vi "Delete DVR Entry for DeviceID.vi"(10 "DVR Array":refnum<data-value>[](array[refnum]), 11 "DeviceID":T1) -> ()   [LabVIEW 2018]
uses:
  <vilib>/ORNL/CSEISMIC DDS/CSEISMIC DDS Base/Data Types/Controls/DeviceID.ctl
  <vilib>/ORNL/CSEISMIC DDS/CSEISMIC DDS Base/CSEISMIC DDS.lvclass
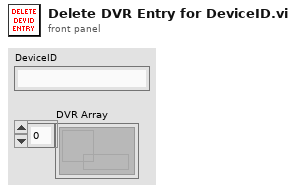
[diagram p1: front panel]
types:
  T1 = typedef "CSEISMIC DDS.lvlib/CSEISMIC DDS.lvclass/DeviceID.ctl" = string
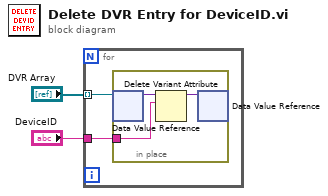
[diagram p0: block diagram]
diagram:
  n1 = for {
    tunnel: "DVR Array" -> [w4] mode=indexing
    tunnel: "DeviceID" -> [w3]
    n2 = in-place {
      in-place-border: w3 -> [w6]
      n3 = in-place-dvr #1(w4) -> (w7:variant)  [unwired: 1 out]
      n4 = Delete Variant Attribute(6:w6, 7:w7) -> (3:w5:variant)  [unwired: 1 in, 2 out]
      n5 = in-place-dvr #1(w5) -> ()  [unwired: 2 out]
    }
  }
